vi "Process.vi"(8 "error in":errorcluster, 11 "ParseVectorFile":refnum<class "ParseVectorFile.lvclass">) -> (0 "error out":errorcluster, 3 "ParseVectorFile out":refnum<class "ParseVectorFile.lvclass">)   [LabVIEW 2019, in "ParseVectorFile.lvclass"]
doc: "---------------------------------------------------------------\nJKI State Machine Objects™\nhttp://jki.net/state-machine-objects/\nCopyright (C) 2005-2015, JKI <info@jki.net>\nALL RIGHTS RESERVED"
uses:
  ParseVectorFile.lvclass
  C:/Program Files (x86)/National Instruments/LabVIEW 2019/vi.lib/JKI/JKI SMO/SMO/SMO.lvclass
  <vilib>/JKI/JKI SMO/SMO/Typedefs/Parent Call--Enum.ctl
  Typedefs/PublicEvents--ParseVectorFile.ParsedData.ctl
  ParsePaths/Path.lvclass
  Rectangle/Rectangle.lvclass
  Image/SVGImage.lvclass
  Dot/Dot.lvclass
  <vilib>/JKI/JKI SMO/SMO/SMO.lvclass/SMO.ctl
  ParseVectorFile.lvclass/ParseVectorFile.ctl
  <vilib>/JKI/JKI SMO/SMO/Private/ReftoDVR--SMO.vi
  <vilib>/JKI/JKI SMO/SMO/SMO.lvclass
panel:
  # "For instructions on how to use the JKI State Machine Objects, examples and video tutorials, visit:\nhttp://jki.net/state-machine-objects/\n\nJKI State Machine Objects™\nhttp://jki.net/state-machine-objects/\nCopyright (C) 2005-2015, JKI <info@jki.net>\nALL RIGHTS RESERVED"
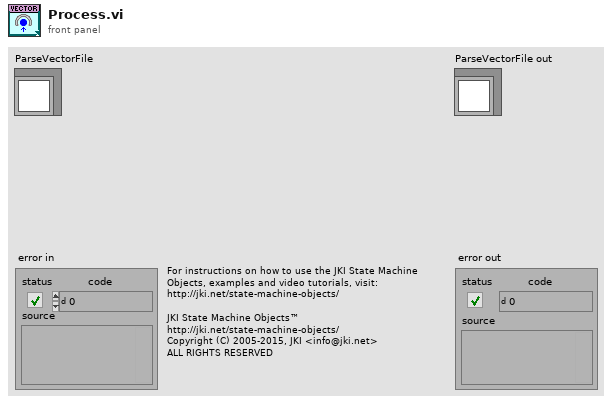
[diagram p1: front panel]
types:
  T1 = typedef "SMO.lvclass/Parent Call--Enum.ctl" = enum16{"Allows parent to run", "Does not request parent to run"}
  T2 = enum32{"invalid app kind", "Development System", "Run Time System", "Student Edition", "Embedded LabVIEW", "Evaluation", "Custom"}
  T3 = enum32{"Invalid", "Standard", "Closed", "Hidden", "Minimized", "Maximized"}
  T4 = enum32{"Bad", "Idle", "Run top level", "Running"}
  T5 = typedef "ParseVectorFile.lvclass/PublicEvents--ParseVectorFile.ParsedData.ctl" = cluster{"Paths":refnum<class "Path.lvclass">[], "Rectangles":refnum<class "Rectangle.lvclass">[], "SVGImage":refnum<class "SVGImage.lvclass">, "Dots":refnum<class "Dot.lvclass">[]}
  T6 = typedef "ParseVectorFile.lvclass/PrivateEvents--ParseVectorFile.NewFile.ctl" = path
  T7 = cluster{"Core":cluster{"Current VI Reference":refnum<vi>, "Close Panel on Exit?":bool, "error":errorcluster}, "Path":path, "Self":refnum<class "ParseVectorFile.lvclass">, "Parsed Data Return":refnum<notifier>, "Last Changed":timestamp}
  T8 = cluster{"Current VI Reference":refnum<vi>, "Close Panel on Exit?":bool, "error":errorcluster}
  T9 = typedef "SMO.lvclass/Protected Events.ctl" = cluster{"StopProcesses":refnum<user-event>, "AbortProcesses":refnum<user-event>, "Config Changed":refnum<user-event>, "Dependency":refnum<user-event>}
  T10 = typedef "ParseVectorFile.lvclass/PrivateEvents--Cluster.ctl" = cluster{"NewFile Asynchronous":refnum<user-event>, "New File Synchronous":refnum<user-event>}
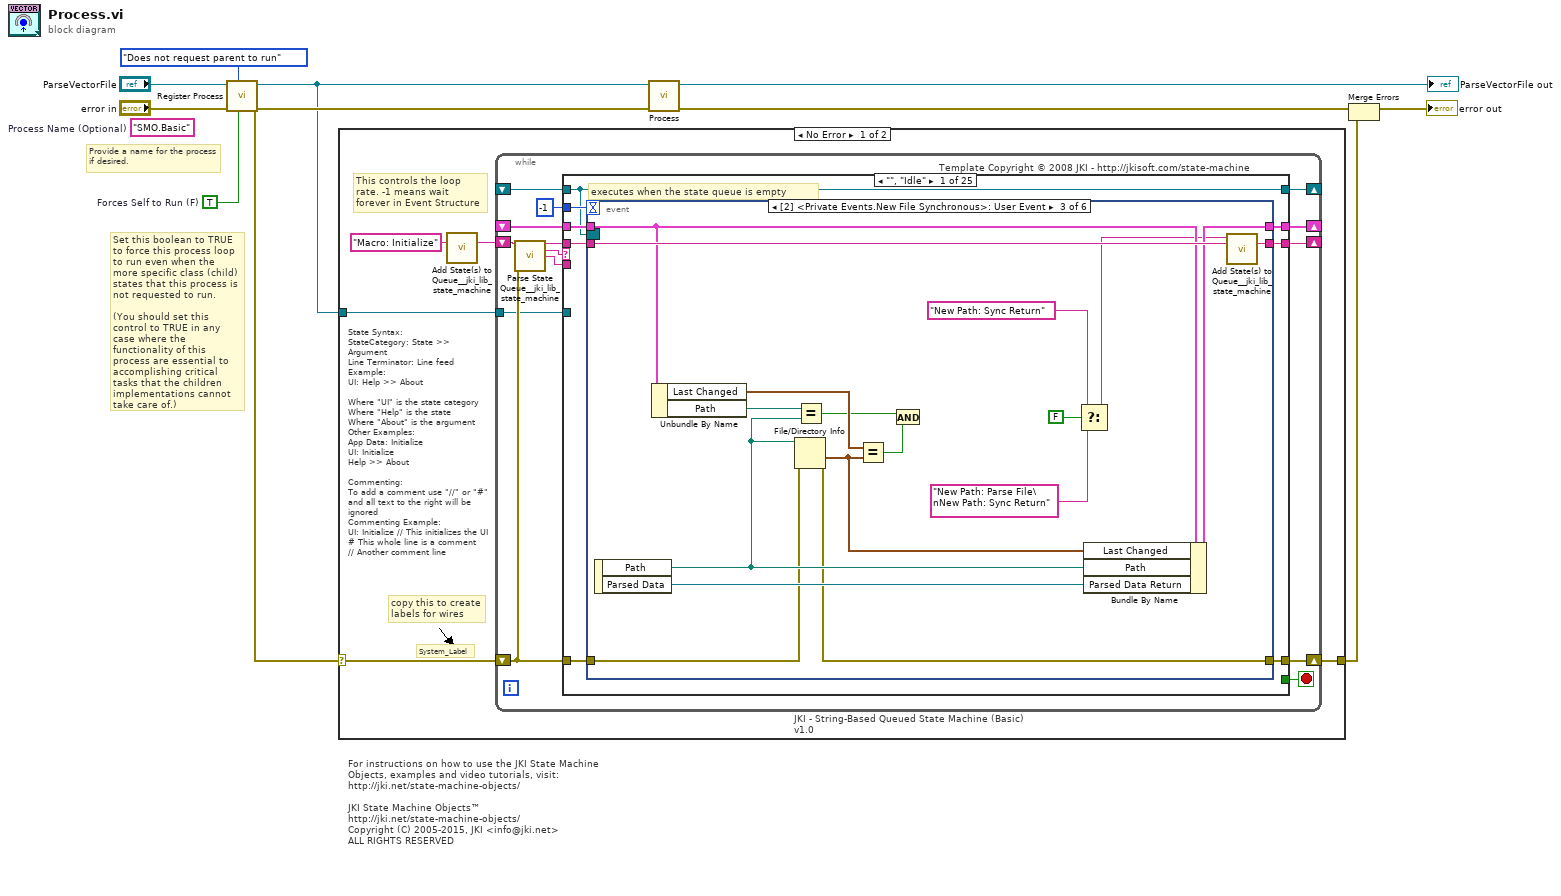
[diagram p0: block diagram]
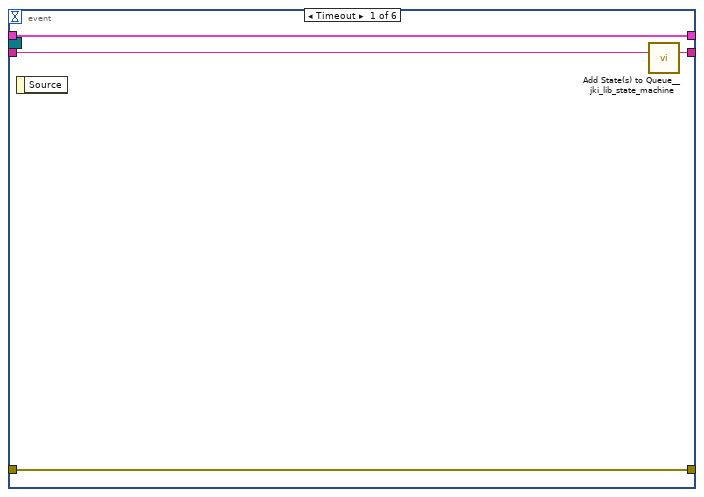
[diagram p2: hidden frame]
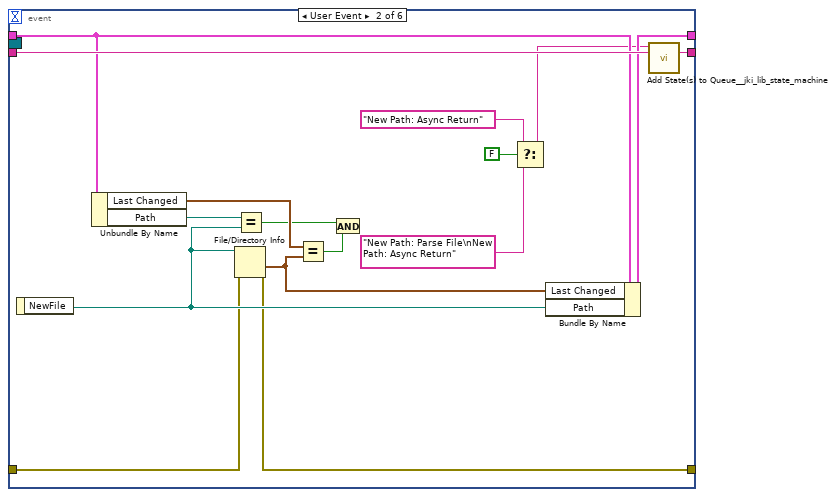
[diagram p3: hidden frame]
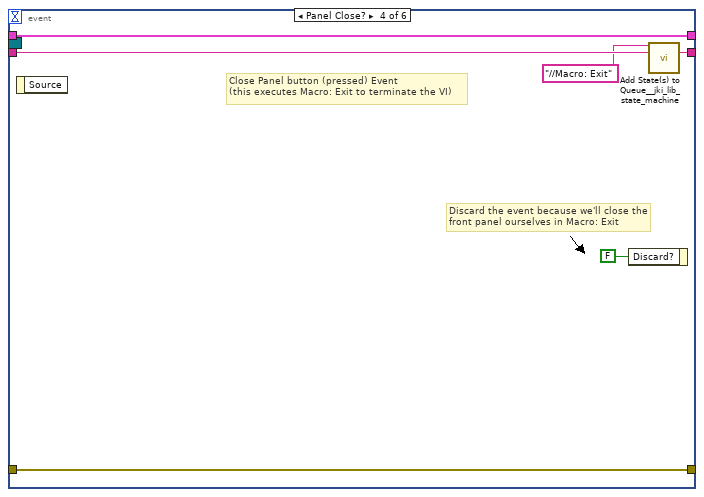
[diagram p4: hidden frame]
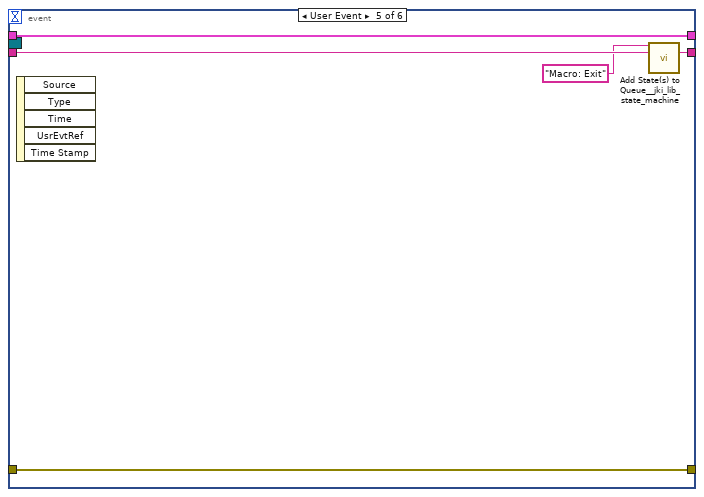
[diagram p5: hidden frame]
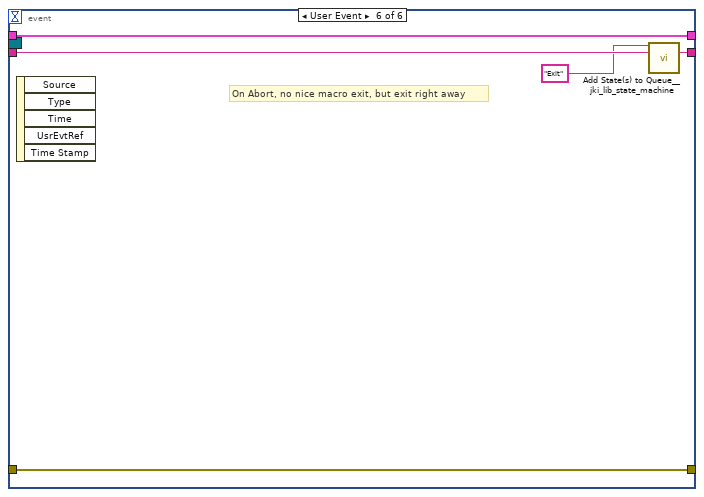
[diagram p6: hidden frame]
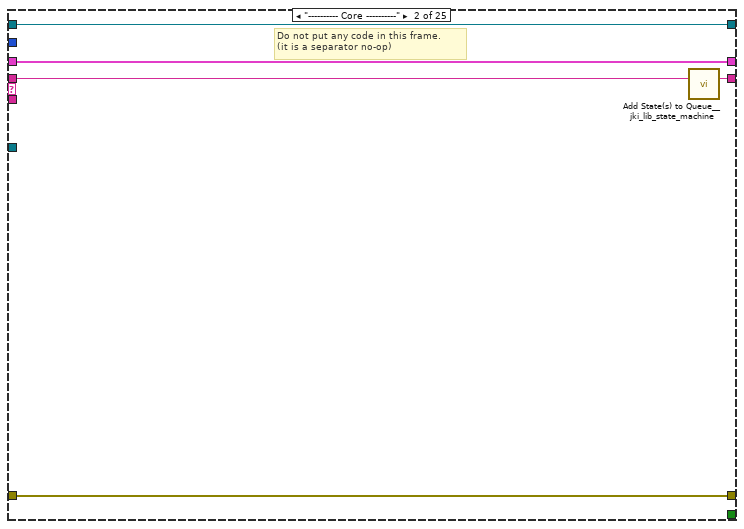
[diagram p7: hidden frame]
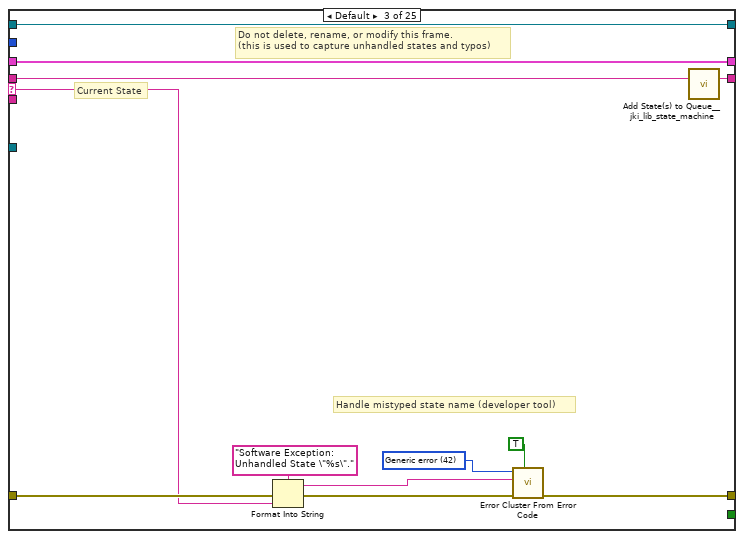
[diagram p8: hidden frame]
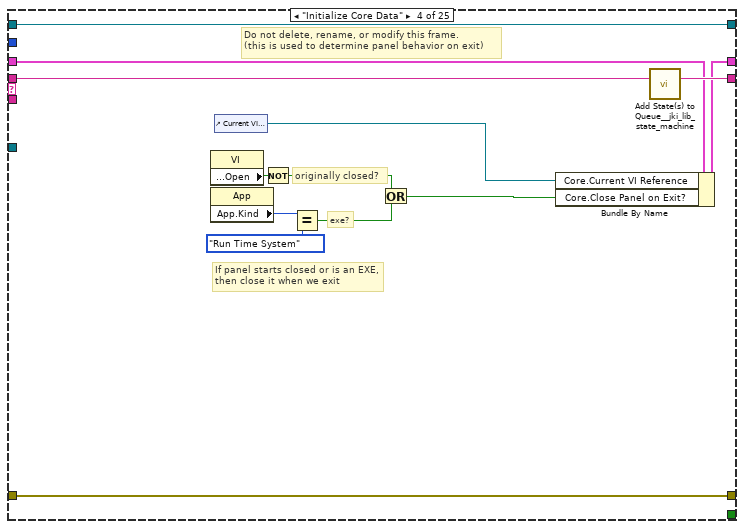
[diagram p9: hidden frame]
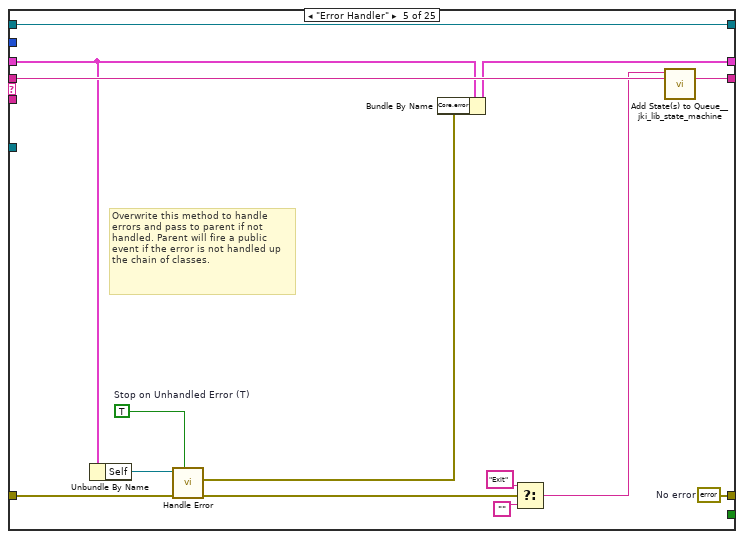
[diagram p10: hidden frame]
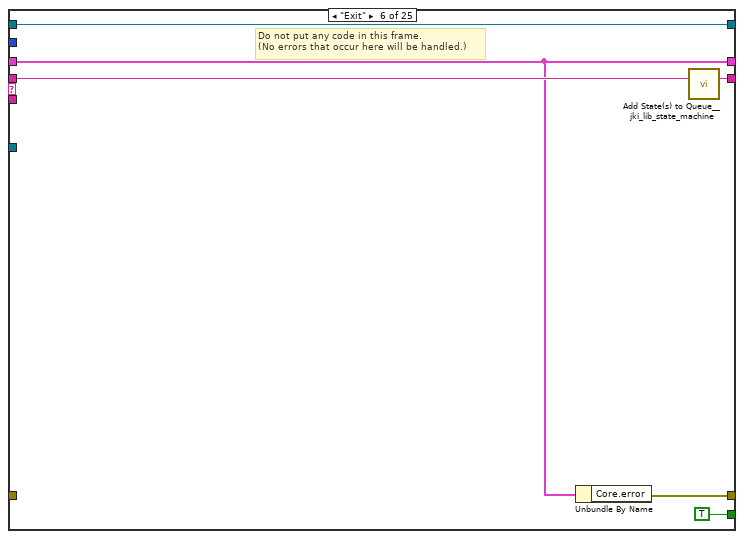
[diagram p11: hidden frame]
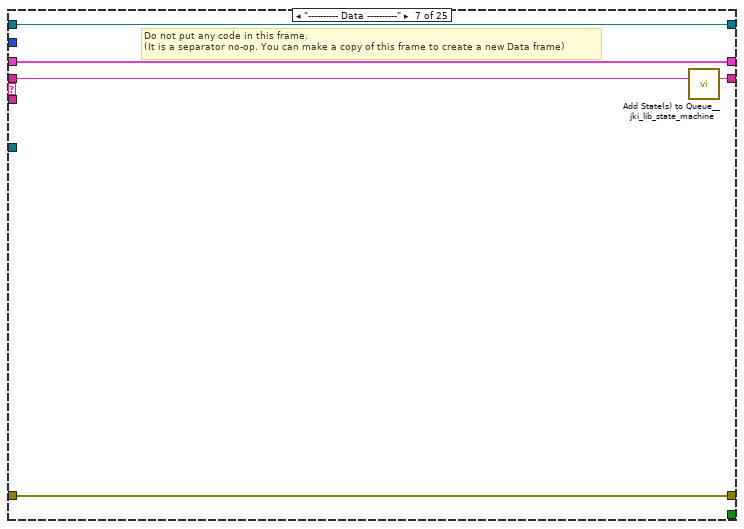
[diagram p12: hidden frame]
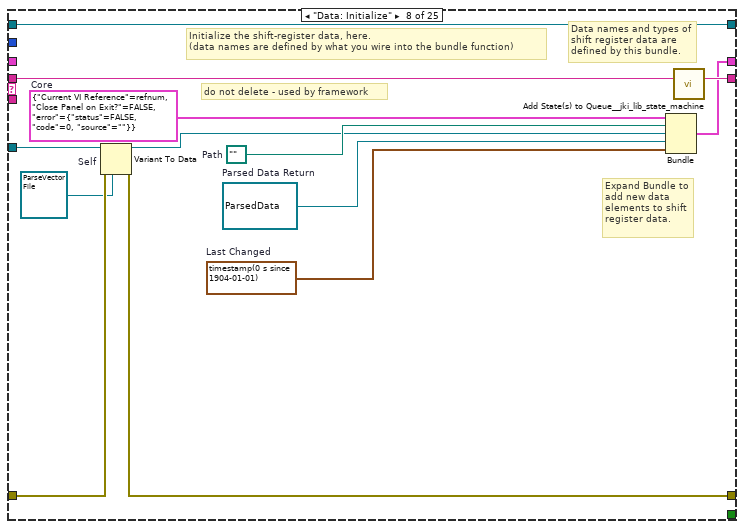
[diagram p13: hidden frame]
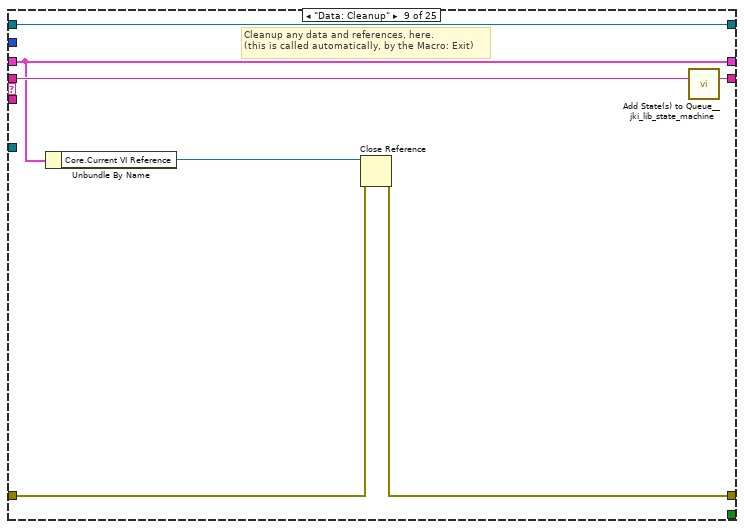
[diagram p14: hidden frame]
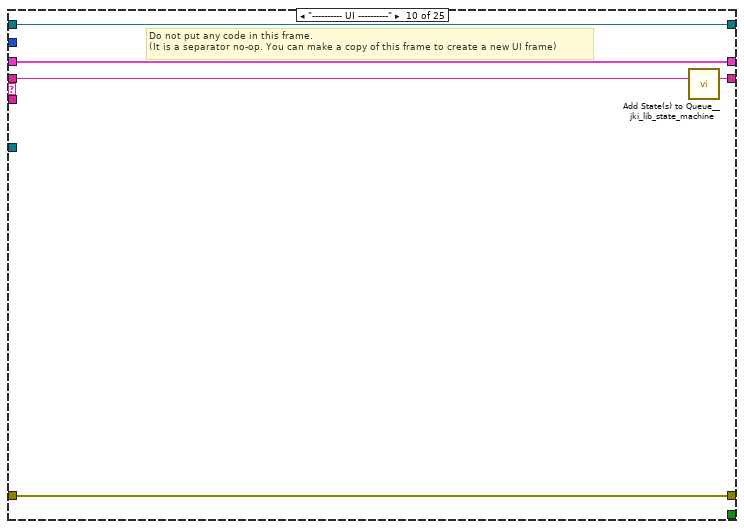
[diagram p15: hidden frame]
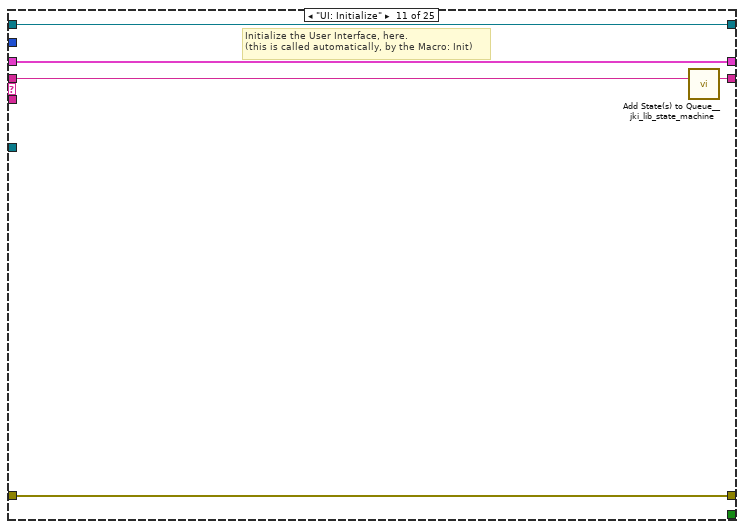
[diagram p16: hidden frame]
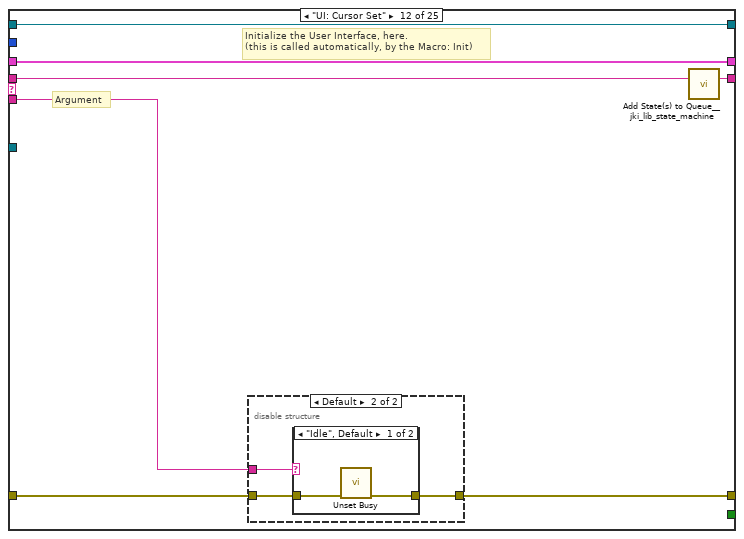
[diagram p17: hidden frame]
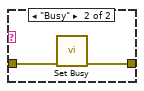
[diagram p19: hidden frame]
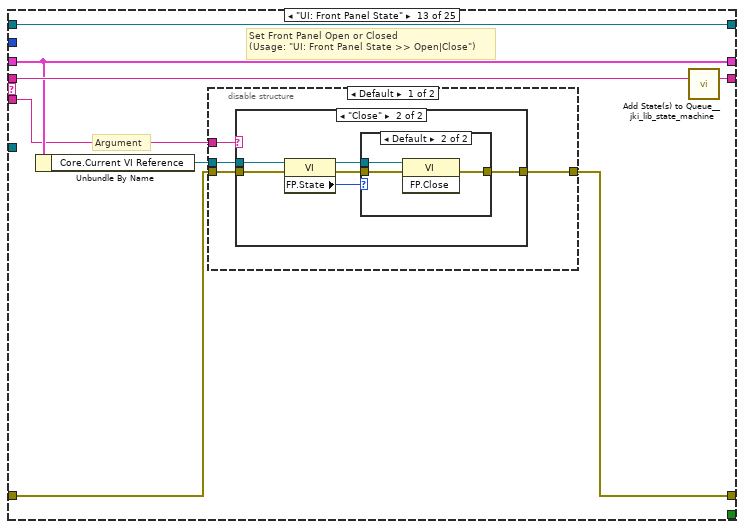
[diagram p20: hidden frame]
diagram:
  w1 = TRUE  # Forces Self to Run (F)
  (unwired) "SMO.Basic"  # Process Name (Optional)
  # "Provide a name for the process\nif desired."
  # "Set this boolean to TRUE to force this process loop to run even when the more specific class (child) states that this process is not requested to run.\n\n(You should set this control to TRUE in any case where the functionality of this process are essential to accomplishing critical tasks that the children implementations cannot take care of.)"
  # "For instructions on how to use the JKI State Machine Objects, examples and video tutorials, visit:\nhttp://jki.net/state-machine-objects/\n\nJKI State Machine Objects™\nhttp://jki.net/state-machine-objects/\nCopyright (C) 2005-2015, JKI <info@jki.net>\nALL RIGHTS RESERVED"
  n1 = call <vilib>:"Register Process.vi"("Forces Self to Run (F)"=w1, "Parent Call"=Parent_Call--Enum."Does not request parent to run", "error in (no error)"="error in", "SMO"="ParseVectorFile") -> ("error out"=w7:errorcluster, "SMO out"=w6:refnum<class "ParseVectorFile.lvclass">)  [unwired: 6 in]
  n2 = case shown="No Error" w7 {
    selector: w7 -> [w12 w345]
    tunnel: w6 -> [w13 _]
    tunnel: [w11 w345] -> w3
    frame No Error {
      # "State Syntax:\nStateCategory: State >> Argument\nLine Terminator: Line feed\nExample:\nUI: Help >> About\n\nWhere \"UI\" is the state category\nWhere \"Help\" is the state\nWhere \"About\" is the argument\nOther Examples:\nApp Data: Initialize\nUI: Initialize\nHelp >> About\n\nCommenting:\nTo add a comment use \"//\" or \"#\" and all text to the right will be ignored\nCommenting Example:\nUI: Initialize // This initializes the UI\n# This whole line is a comment\n// Another comment line"
      # "copy this to create labels for wires"
      # "This controls the loop rate. -1 means wait forever in Event Structure"
      # "System_Label"
      n3 = call <vilib>:"Add State(s) to Queue__jki_lib_state_machine.vi"("State(s) in (\"\")"="Macro: Initialize") -> ("States Out"=w15:string)  [unwired: 14 in]
      n4 = while "JKI - String-Based Queued State Machine (Basic) v1.0" {
        shift-right: [w22] -> _
        shift-left: _ -> [w21]
        shift-right: [w25] -> w11
        shift-left: w12 -> [w19]
        shift-right: [w24] -> _
        shift-left: w15 -> [w26]
        tunnel: w13 -> [w18]
        shift-right: [w17] -> _
        shift-left: _ -> [w16]
        stop <- w23 stop-if-true
        # "Template Copyright © 2008 JKI - http://jkisoft.com/state-machine"
        n5 = call <vilib>:"Parse State Queue__jki_lib_state_machine.vi"("State Queue"=w26, "Error In (no error)"=w19) -> ("Remaining States"=w28:string, "Current State"=w29:string, "Arguments"=w27:string)  [unwired: 11 in]
        n6 = case shown="\"\", \"Idle\"" w29 {
          selector: w29 -> [_ _ w97 _ _ _ _ _ _ _ _ _ _ _ _ _ _ _ _ _ _ _ _ _ _]
          tunnel: w28 -> [w37 w95 w101 w120 w134 w140 w145 w158 w165 w170 w175 w182 w198 w230 w244 w258 w263 w274 w279 w291 w297 w304 w319 w334 w344]
          tunnel: w27 -> [_ _ _ _ _ _ _ _ _ _ _ w176 w192 _ _ _ _ _ _ _ _ _ _ _ _]
          tunnel: w21 -> [w35 w92 w99 w111 w128 w136 w142 _ w160 w167 w173 w180 w194 w227 w240 w249 w260 w271 w276 w289 w295 w299 w315 w330 w341]
          tunnel: [w34 w93 w103 w117 w129 w135 w143 w154 w161 w168 w172 w177 w195 w228 w242 w256 w261 w265 w277 w285 w293 w301 w307 w322 w335] -> w25
          tunnel: w19 -> [w33 w93 w102 w117 w130 _ w143 w155 w162 w168 w172 w178 w196 w228 w242 w256 w261 w266 w277 w286 w293 w301 w307 w321 w338]
          tunnel: [w36 w94 w100 w119 w133 w139 w144 w157 w164 w169 w174 w181 w197 w229 w243 w257 w262 w273 w278 w290 w296 w303 w318 w333 w343] -> w24
          tunnel: [_ _ _ _ _ TRUE _ _ _ _ _ _ _ _ _ _ _ _ _ _ _ _ _ _ _] -> w23
          tunnel: [w32 w92 w99 w118 w127 w136 w142 w156 w160 w167 w173 w180 w194 w227 w240 w249 w260 w271 w276 w289 w295 w300 w316 w331 w340] -> w22
          tunnel: -1 ("Timeout") -> [w31 _ _ _ _ _ _ _ _ _ _ _ _ _ _ _ _ _ _ _ _ _ _ _ _]
          tunnel: w18 -> [_ _ _ _ _ _ _ w153 _ _ _ _ _ _ _ _ _ _ _ _ _ _ _ _ _]
          tunnel: [w30 w91 w96 w108 w132 w137 w141 w152 w159 w166 w171 w179 w191 w226 w241 w250 w259 w272 w275 w288 w294 w302 w317 w332 w342] -> w17
          tunnel: w16 -> [w30 w91 w96 w108 w132 w137 w141 w152 w159 w166 w171 w179 w191 w226 w241 w250 w259 w272 w275 _ w294 w302 w317 w332 w342]
          frame "", "Idle" {
            # "executes when the state queue is empty"
            n7 = event shown="[2] <Private Events.New File Synchronous>: User Event" {
              selector: w30 -> [_ _ _ _ _ _]
              dyn-events: _ -> [_ _ _ _ _ _]
              timeout: w31 -> [_ _ _ _ _ _]
              tunnel: w37 -> [w41 w57 w74 w80 w85 w90]
              tunnel: [w40 w56 w73 w79 w84 w89] -> w36
              tunnel: w35 -> [w39 w54 w65 w77 w82 w87]
              tunnel: [w38 w51 w60 w78 w83 w88] -> w34
              tunnel: w33 -> [w38 w50 w59 w78 w83 w88]
              tunnel: [w39 w55 w72 w77 w82 w87] -> w32
              event Timeout {
                n8 = event-data() -> ()  [unwired: 1 in, 1 out]
                n9 = call <vilib>:"Add State(s) to Queue__jki_lib_state_machine.vi"("State(s) in (\"\")"=w41) -> ("States Out"=w40:string)  [unwired: 14 in]
              }
              event User Event {
                n10 = event-data() -> ("NewFile"=w52:T6)  [unwired: 1 in]
                n11 = Unbundle By Name(w54) -> ("Last Changed"=w49:timestamp, "Path"=w53:path)
                n12 = File/Directory Info(path=w52, error in=w50) -> (last mod=w46:timestamp, error out=w51:errorcluster)  [unwired: 5 out]
                n13 = Equal?(x=w53, y=w52) -> (x = y?=w48:bool)
                n14 = Equal?(x=w49, y=w46) -> (x = y?=w47:bool)
                n15 = And(x=w48, y=w47) -> ()  [unwired: 1 out]
                n16 = Select(t="New Path: Async Return", s=FALSE, f="New Path: Parse File\nNew Path: Async Return") -> (s? t:f=w43:string)
                n17 = Bundle By Name(cluster=w54, "Last Changed"=w46, "Path"=w52) -> (w55:T7)
                n18 = call <vilib>:"Add State(s) to Queue__jki_lib_state_machine.vi"("State(s) in Front (\"\")"=w43, "State(s) in (\"\")"=w57) -> ("States Out"=w56:string)  [unwired: 13 in]
              }
              event User Event {
                n19 = event-data() -> ("Path"=w64:path, "Parsed Data"=w71:refnum<notifier>)  [unwired: 1 in]
                n20 = Unbundle By Name(w65) -> ("Last Changed"=w69:timestamp, "Path"=w70:path)
                n21 = File/Directory Info(path=w64, error in=w59) -> (last mod=w63:timestamp, error out=w60:errorcluster)  [unwired: 5 out]
                n22 = Equal?(x=w70, y=w64) -> (x = y?=w68:bool)
                n23 = Equal?(x=w69, y=w63) -> (x = y?=w67:bool)
                n24 = And(x=w68, y=w67) -> ()  [unwired: 1 out]
                n25 = Select(t="New Path: Sync Return", s=FALSE, f="New Path: Parse File\nNew Path: Sync Return") -> (s? t:f=w61:string)
                n26 = Bundle By Name(cluster=w65, "Last Changed"=w63, "Path"=w64, "Parsed Data Return"=w71) -> (w72:T7)
                n27 = call <vilib>:"Add State(s) to Queue__jki_lib_state_machine.vi"("State(s) in Front (\"\")"=w61, "State(s) in (\"\")"=w74) -> ("States Out"=w73:string)  [unwired: 13 in]
              }
              event Panel Close? {
                # "Discard the event because we'll close the front panel ourselves in Macro: Exit"
                # "Close Panel button (pressed) Event\n(this executes Macro: Exit to terminate the VI)"
                n28 = event-data() -> ()  [unwired: 1 in, 1 out]
                n29 = event-data("Discard?"=FALSE) -> ()  [unwired: 1 in, 1 out]
                n30 = call <vilib>:"Add State(s) to Queue__jki_lib_state_machine.vi"("State(s) in Front (\"\")"="//Macro: Exit", "State(s) in (\"\")"=w80) -> ("States Out"=w79:string)  [unwired: 13 in]
              }
              event User Event {
                n31 = event-data() -> ()  [unwired: 1 in, 5 out]
                n32 = call <vilib>:"Add State(s) to Queue__jki_lib_state_machine.vi"("State(s) in Front (\"\")"="Macro: Exit", "State(s) in (\"\")"=w85) -> ("States Out"=w84:string)  [unwired: 13 in]
              }
              event User Event {
                # "On Abort, no nice macro exit, but exit right away"
                n33 = event-data() -> ()  [unwired: 1 in, 5 out]
                n34 = call <vilib>:"Add State(s) to Queue__jki_lib_state_machine.vi"("State(s) in Front (\"\")"="Exit", "State(s) in (\"\")"=w90) -> ("States Out"=w89:string)  [unwired: 13 in]
              }
            }
          }
          frame "---------- Core ----------" {
            # "Do not put any code in this frame.\n(it is a separator no-op)"
            n35 = call <vilib>:"Add State(s) to Queue__jki_lib_state_machine.vi"("State(s) in (\"\")"=w95) -> ("States Out"=w94:string)  [unwired: 14 in]
          }
          frame Default {
            w106 = 42 items=["No error", "Argument error", "Memory is full", "Out of zone", "End of file", "File already open", "Generic file I/O error", "File not found", "File permission error", "Disk is full", "Duplicate path", "Too many files open", "System feature not enabled", "Resource file not found", "Cannot add resource", "Resource not found", "Image not found", "Image memory error", "Pen does not exist", "Config type invalid", "Config token not found", "Config parse error", "Config memory error", "Bad external code format", "Bad external code offset", "External code not present", "Null window", "Destroy window error", "Null menu", "Print aborted", "Bad print record", "Print driver error", "Windows error during printing", "Memory error during printing", "Print dialog error", "Generic print error", "Invalid device refnum", "Device not found", "Device parameter error", "Device unit error", "Cannot open device", "Device call aborted", "Generic error", "Cancelled by user", "Object ID too low", "Object ID too high", "Object not in heap", "Unknown heap", "Unknown object (invalid DefProc)", "Unknown object (DefProc not in table)", "Message out of range", "Invalid (null) method", "Unknown message", "Manager call not supported", "Bad address", "Network operation in progress", "Network operation timed out", "Connection is busy", "Network attribute not supported", "Network error", "Address in use", "System out of memory", "Connection aborted", "Connection refused", "Not connected", "Already connected", "Connection closed", "Initialization error (interapplication manager)", "Bad occurrence", "Wait on unbound occurrence handler", "Occurrence queue overflow", "Datalog type conflict", "Unused", "Unrecognized type (interapplication manager)", "Memory corrupt", "Failed to make temporary DLL", "Old CIN version", "Drag socket not found", "Failed to load drop-object", "Failed to register OLE object", "Failed to release OLE object", "Format specifier type mismatch", "Unknown format specifier", "Too few format specifiers", "Too many format specifiers", "Scan failed", "Newer CIN version", "Error converting to variant", "Runtime menu error", "Password tampered", "Variant attribute not found", "Incompatible variant data type", "Event data is not available", "Event Store is not present", "Occurrence is not found", "Event Queue is not created", "Event info is not available", "Refnum passed is NULL", "Error retrieving Class GUID", "Error retrieving CoClass GUID", "Error retrieving TypeLib GUID.", "Bad built application magic bytes.", "Specific driver is different from the specific driver associated with the Logical Name.", "There is no session opened to the class driver.", "Max Error", "MAX - Error with config objects", "MAX - Error loading configuration", "MAX - Group not supported"]
            # "Current State"
            # "Do not delete, rename, or modify this frame.\n(this is used to capture unhandled states and typos)"
            # "Handle mistyped state name (developer tool)"
            n36 = Format Into String(format string="Software Exception: Unhandled State \"%s\"." ("message"), error in=w102, w97) -> (resulting string=w105:string, error out=w104:errorcluster)  [unwired: 1 in]
            n37 = call <vilib>:"Error Cluster From Error Code.vi"("show call chain? (False)"=TRUE, "error in (no error)"=w104, "error message (\"\")"=w105, "error code (0)"=w106) -> ("error out"=w103:errorcluster)  [unwired: 5 in]
            n38 = call <vilib>:"Add State(s) to Queue__jki_lib_state_machine.vi"("State(s) in (\"\")"=w101) -> ("States Out"=w100:string)  [unwired: 14 in]
          }
          frame "Initialize Core Data" {
            # "Do not delete, rename, or modify this frame.\n(this is used to determine panel behavior on exit)"
            # "originally closed?"
            # "exe?"
            # "If panel starts closed or is an EXE, then close it when we exit"
            n39 = property class="VI"() -> ("Front Panel.Open"=w116:bool)  [unwired: 2 in, 2 out]
            n40 = property class="App"() -> ("App.Kind"=w115:T2)  [unwired: 2 in, 2 out]
            n41 = control-ref of="Current VI Reference"() -> (w109:refnum<vi>)
            n42 = Not(x=w116) -> (.not. x?=w113:bool)
            n43 = Equal?(x=w115, y=T2."Run Time System" ("Application:Kind")) -> (x = y?=w112:bool)
            n44 = Or(x=w113, y=w112) -> (x .or. y?=w110:bool)
            n45 = Bundle By Name(cluster=w111, "Core.Current VI Reference"=w109, "Core.Close Panel on Exit?"=w110) -> (w118:T7)
            n46 = call <vilib>:"Add State(s) to Queue__jki_lib_state_machine.vi"("State(s) in (\"\")"=w120) -> ("States Out"=w119:string)  [unwired: 14 in]
          }
          frame "Error Handler" {
            w121 = TRUE  # Stop on Unhandled Error (T)
            w129 = errorcluster {"status"=FALSE, "code"=0, "source"=""}  # No error
            # "Overwrite this method to handle errors and pass to parent if not handled. Parent will fire a public event if the error is not handled up the chain of classes."
            n47 = Unbundle By Name(w128) -> ("Self"=w131:refnum<class "ParseVectorFile.lvclass">)
            n48 = call-dynamic "Handle Error.vi"("Stop on Unhandled Error (T)"=w121, "error in"=w130, "SMO"=w131) -> ("handling error"=w122:errorcluster, "Unhandled error"=w125:errorcluster)  [unwired: 6 in, 1 out]
            n49 = Bundle By Name(cluster=w128, "Core.error"=w125) -> (w127:T7)
            n50 = Select(t="Exit", s=w122, f="") -> (s? t:f=w126:string)
            n51 = call <vilib>:"Add State(s) to Queue__jki_lib_state_machine.vi"("State(s) in Front (\"\")"=w126, "State(s) in (\"\")"=w134) -> ("States Out"=w133:string)  [unwired: 13 in]
          }
          frame "Exit" {
            # "Do not put any code in this frame.\n(No errors that occur here will be handled.)"
            n52 = Unbundle By Name(w136) -> ("Core.error"=w135:errorcluster)
            n53 = call <vilib>:"Add State(s) to Queue__jki_lib_state_machine.vi"("State(s) in (\"\")"=w140) -> ("States Out"=w139:string)  [unwired: 14 in]
          }
          frame "---------- Data ----------" {
            # "Do not put any code in this frame.\n(It is a separator no-op. You can make a copy of this frame to create a new Data frame)"
            n54 = call <vilib>:"Add State(s) to Queue__jki_lib_state_machine.vi"("State(s) in (\"\")"=w145) -> ("States Out"=w144:string)  [unwired: 14 in]
          }
          frame "Data: Initialize" {
            w146 = timestamp(0 s since 1904-01-01)  # Last Changed
            w149 = refnum<notifier> refnum  # Parsed Data Return
            w150 = path ""  # Path
            w151 = T8 {"Current VI Reference"=refnum, "Close Panel on Exit?"=FALSE, "error"={"status"=FALSE, "code"=0, "source"=""}}  # Core
            w148 = refnum<class "ParseVectorFile.lvclass"> refnum  # Self
            # "do not delete - used by framework"
            # "Expand Bundle to add new data elements to shift register data."
            # "Data names and types of shift register data are defined by this bundle."
            # "Initialize the shift-register data, here.\n(data names are defined by what you wire into the bundle function)"
            n55 = Variant To Data(error in=w155, type=w148, Variant=w153) -> (data=w147:refnum<class "ParseVectorFile.lvclass">, error out=w154:errorcluster)
            n56 = Bundle("Core"=w151, "Path"=w150, "Self"=w147, "Parsed Data Return"=w149, "Last Changed"=w146) -> (w156:T7)  [unwired: 1 in]
            n57 = call <vilib>:"Add State(s) to Queue__jki_lib_state_machine.vi"("State(s) in (\"\")"=w158) -> ("States Out"=w157:string)  [unwired: 14 in]
          }
          frame "Data: Cleanup" {
            # "Cleanup any data and references, here.\n(this is called automatically, by the Macro: Exit)"
            n58 = Unbundle By Name(w160) -> ("Core.Current VI Reference"=w163:refnum<vi>)
            n59 = Close Reference(reference=w163, error in (no error)=w162) -> (error out=w161:errorcluster)
            n60 = call <vilib>:"Add State(s) to Queue__jki_lib_state_machine.vi"("State(s) in (\"\")"=w165) -> ("States Out"=w164:string)  [unwired: 14 in]
          }
          frame "---------- UI ----------" {
            # "Do not put any code in this frame.\n(It is a separator no-op. You can make a copy of this frame to create a new UI frame)"
            n61 = call <vilib>:"Add State(s) to Queue__jki_lib_state_machine.vi"("State(s) in (\"\")"=w170) -> ("States Out"=w169:string)  [unwired: 14 in]
          }
          frame "UI: Initialize" {
            # "Initialize the User Interface, here.\n(this is called automatically, by the Macro: Init)"
            n62 = call <vilib>:"Add State(s) to Queue__jki_lib_state_machine.vi"("State(s) in (\"\")"=w175) -> ("States Out"=w174:string)  [unwired: 14 in]
          }
          frame "UI: Cursor Set" {
            # "Argument"
            # "Initialize the User Interface, here.\n(this is called automatically, by the Macro: Init)"
            n63 = disable-structure shown="Default" {
              disable-tunnel: w178 -> [w183 w186]
              disable-tunnel: [w183 w185] -> w177
              disable-tunnel: w176 -> [_ w184]
              frame condition #0 {
              }
              frame condition #1 (active) {
                n64 = case shown="\"Idle\", Default" w184 {
                  tunnel: w186 -> [w188 w190]
                  tunnel: [w187 w189] -> w185
                  frame "Idle", Default {
                    n65 = call <vilib>:"Unset Busy.vi"("error in (no error)"=w188) -> ("error out"=w187:errorcluster)  [unwired: 10 in]
                  }
                  frame "Busy" {
                    n66 = call <vilib>:"Set Busy.vi"("error in (no error)"=w190) -> ("error out"=w189:errorcluster)  [unwired: 9 in, 1 out]
                  }
                }
              }
            }
            n67 = call <vilib>:"Add State(s) to Queue__jki_lib_state_machine.vi"("State(s) in (\"\")"=w182) -> ("States Out"=w181:string)  [unwired: 14 in]
          }
          frame "UI: Front Panel State" {
            # "Argument"
            # "Set Front Panel Open or Closed\n(Usage: \"UI: Front Panel State >> Open|Close\")"
            n68 = Unbundle By Name(w194) -> ("Core.Current VI Reference"=w193:refnum<vi>)
            n69 = disable-structure shown="Default" {
              disable-tunnel: w196 -> [w202 w225]
              disable-tunnel: [w201 w225] -> w195
              disable-tunnel: w193 -> [w200 _]
              disable-tunnel: w192 -> [w199 _]
              frame condition #0 (active) {
                n70 = case shown="\"Close\"" w199 {
                  tunnel: w202 -> [w206 w219]
                  tunnel: [w208 w220] -> w201
                  tunnel: w200 -> [w207 w217]
                  frame "Open", Default {
                    n71 = property class="VI"(reference=w207, error in=w206) -> (reference out=w204:refnum<vi>, error out=w205:errorcluster, "FP.State"=w203:T3)
                    n72 = case shown="\"Closed\"" w203 {
                      tunnel: [w211 w214] -> w208
                      tunnel: w205 -> [w210 w214]
                      tunnel: w204 -> [w209 _]
                      frame "Closed" {
                        n73 = invoke class="VI" method="FP.Open"(reference=w209, error in=w210, "Activate"=TRUE, "State"=T3."Standard") -> (error out=w211:errorcluster)  [unwired: 1 in, 4 out]
                      }
                      frame Default {
                      }
                    }
                  }
                  frame "Close" {
                    n74 = property class="VI"(reference=w217, error in=w219) -> (reference out=w216:refnum<vi>, error out=w218:errorcluster, "FP.State"=w215:T3)
                    n75 = case shown="Default" w215 {
                      tunnel: [w221 w224] -> w220
                      tunnel: w218 -> [w221 w223]
                      tunnel: w216 -> [_ w222]
                      frame "Invalid", "Closed" {
                      }
                      frame Default {
                        n76 = invoke class="VI" method="FP.Close"(reference=w222, error in=w223) -> (error out=w224:errorcluster)  [unwired: 1 in, 2 out]
                      }
                    }
                  }
                }
              }
              frame condition #1 {
              }
            }
            n77 = call <vilib>:"Add State(s) to Queue__jki_lib_state_machine.vi"("State(s) in (\"\")"=w198) -> ("States Out"=w197:string)  [unwired: 14 in]
          }
          frame "---------- Macro ----------" {
            # "Do not put any code in this frame.\n(It is a separator no-op. You can make a copy of this frame to create a new Macro frame)"
            n78 = call <vilib>:"Add State(s) to Queue__jki_lib_state_machine.vi"("State(s) in (\"\")"=w230) -> ("States Out"=w229:string)  [unwired: 14 in]
          }
          frame "Macro: Initialize" {
            w235 = "//UI: Initialize\n//UI: Front Panel State >> Open"  # //UI: Initialize //UI: Front Panel State >> Open
            w231 = "Process: Sync"
            # "Initialization Macro\n(This is called once, when the VI starts)"
            n79 = control-ref of="This VI"() -> (w233:refnum<vi>)
            n80 = property class="VI"(reference=w233) -> ("Exec.State"=w232:T4)  [unwired: 1 in, 2 out]
            n81 = Equal?(x=w232, y=T4."Run top level") -> (x = y?=w238:bool)
            n82 = Select(t=w231, s=w238, f="") -> ()  [unwired: 1 out]
            n83 = call <vilib>:"Add State(s) to Queue__jki_lib_state_machine.vi"("State(s) in Front (\"\")"="Data: Initialize\nInitialize Core Data\nEvents: Register", "State(s) in (\"\")"=w231, "State(s) at Back (\"\")"=w235) -> ("States Out"=w234:string)  [unwired: 12 in]
            n84 = call <vilib>:"Add State(s) to Queue__jki_lib_state_machine.vi"("State(s) in Front (\"\")"=w234, "State(s) in (\"\")"=w244) -> ("States Out"=w243:string)  [unwired: 13 in]
          }
          frame "Macro: Exit" {
            # "Exit Macro\n(This is called once, when the VI exits)"
            n85 = Unbundle By Name(w249) -> ("Core.Close Panel on Exit?"=w255:bool)
            n86 = Select(t="UI: Front Panel State >> Close", s=w255, f="") -> (s? t:f=w252:string)
            n87 = call <vilib>:"Add State(s) to Queue__jki_lib_state_machine.vi"("State(s) in Front (\"\")"="Data: Cleanup\nEvents: Unregister", "State(s) in (\"\")"="Process: Sync", "State(s) at Back (\"\")"="Exit") -> ("States Out"=w246:string)  [unwired: 12 in]
            n88 = call <vilib>:"Add State(s) to Queue__jki_lib_state_machine.vi"("State(s) in (\"\")"=w252, "State(s) at Back (\"\")"=w246) -> ("States Out"=w251:string)  [unwired: 13 in]
            n89 = call <vilib>:"Add State(s) to Queue__jki_lib_state_machine.vi"("State(s) in Front (\"\")"=w251, "State(s) in (\"\")"=w258) -> ("States Out"=w257:string)  [unwired: 13 in]
          }
          frame "---------- Process ----------" {
            # "Template Separator\n(You can make a copy of, or modify, this frame)"
            n90 = call <vilib>:"Add State(s) to Queue__jki_lib_state_machine.vi"("State(s) in (\"\")"=w263) -> ("States Out"=w262:string)  [unwired: 14 in]
          }
          frame "Process: Sync" {
            n91 = Unbundle By Name(w271) -> ("Self"=w267:refnum<class "ParseVectorFile.lvclass">)
            n92 = call <vilib>:"WaitOnProcessSync.vi"("error in (no error)"=w266, "SMO"=w267) -> ("error out"=w265:errorcluster, "Don't run?"=w270:bool)  [unwired: 7 in, 1 out]
            n93 = Select(t="Data: Cleanup\nEvents: Unregister\nExit", s=w270, f="") -> (s? t:f=w264:string)
            n94 = call <vilib>:"Add State(s) to Queue__jki_lib_state_machine.vi"("State(s) in Front (\"\")"=w264, "State(s) in (\"\")"=w274) -> ("States Out"=w273:string)  [unwired: 13 in]
          }
          frame "---------- Events ----------" {
            # "Template Separator\n(You can make a copy of, or modify, this frame)"
            n95 = call <vilib>:"Add State(s) to Queue__jki_lib_state_machine.vi"("State(s) in (\"\")"=w279) -> ("States Out"=w278:string)  [unwired: 14 in]
          }
          frame "Events: Register" {
            # "Expand to add\nmore events"
            n96 = Unbundle By Name(w289) -> ("Self"=w282:refnum<class "ParseVectorFile.lvclass">)
            n97 = call <vilib>:"GetProtectedEvents.vi"("SMO"=w282) -> ("error out"=w283:errorcluster, "SMO Protected Events"=w287:T9)  [unwired: 8 in, 1 out]
            n98 = call "ParseVectorFile.GetPrivateEvents.vi"("ParseVectorFile"=w282) -> ("error out"=w281:errorcluster, "Private Events"=w280:T10)  [unwired: 8 in, 1 out]
            n99 = register-events(w287, w280) -> (reference out=w288:refnum<event-registration>, error out=w284:errorcluster)  [unwired: 2 in]
            n100 = Merge Errors(w286, w284, w283, w281) -> (w285:errorcluster)
            n101 = call <vilib>:"Add State(s) to Queue__jki_lib_state_machine.vi"("State(s) in (\"\")"=w291) -> ("States Out"=w290:string)  [unwired: 14 in]
          }
          frame "Events: Unregister" {
            n102 = Unregister For Events(event registration refnum=w294, error in=w293) -> (error out=w292:errorcluster)
            n103 = call <vilib>:"Clear Errors.vi"("error in (no error)"=w292) -> ()  [unwired: 5 in, 2 out]
            n104 = call <vilib>:"Add State(s) to Queue__jki_lib_state_machine.vi"("State(s) in (\"\")"=w297) -> ("States Out"=w296:string)  [unwired: 14 in]
          }
          frame "---------- New Path ----------" {
            n105 = Unbundle By Name(w299) -> ("Path"=w298:path)
            n106 = Bundle By Name(cluster=w299, "Path"=w298) -> (w300:T7)
            n107 = call <vilib>:"Add State(s) to Queue__jki_lib_state_machine.vi"("State(s) in (\"\")"=w304) -> ("States Out"=w303:string)  [unwired: 14 in]
          }
          frame "New Path: Sync Return" {
            n108 = Unbundle By Name(w315) -> ("Parsed Data Return"=w309:refnum<notifier>, "Self"=w306:refnum<class "ParseVectorFile.lvclass">)
            n109 = Unbundle By Name(w306) -> ("Paths"=w313:refnum<class "Path.lvclass">[], "Rectangles"=w312:refnum<class "Rectangle.lvclass">[], "SVGImage"=w311:refnum<class "SVGImage.lvclass">, "Dots"=w305:refnum<class "Dot.lvclass">[])
            n110 = Bundle By Name(cluster=T5 {"Paths"=[], "Rectangles"=[], "SVGImage"=refnum, "Dots"=[]} ("ParsedData"), "Paths"=w313, "Rectangles"=w312, "SVGImage"=w311, "Dots"=w305) -> (w310:T5)
            n111 = Send Notification(notification=w310, notifier=w309) -> (error out=w308:errorcluster)  [unwired: 1 in, 1 out]
            n112 = call <vilib>:"Clear Errors.vi"("error in (no error)"=w308) -> ()  [unwired: 5 in, 2 out]
            n113 = Bundle By Name(cluster=w315, "Self"=w306) -> (w316:T7)
            n114 = call <vilib>:"Add State(s) to Queue__jki_lib_state_machine.vi"("State(s) in (\"\")"=w319) -> ("States Out"=w318:string)  [unwired: 14 in]
          }
          frame "New Path: Async Return" {
            n115 = Unbundle By Name(w330) -> ("Self"=w324:refnum<class "ParseVectorFile.lvclass">)
            n116 = Unbundle By Name(w324) -> ("Paths"=w327:refnum<class "Path.lvclass">[], "Rectangles"=w326:refnum<class "Rectangle.lvclass">[], "SVGImage"=w325:refnum<class "SVGImage.lvclass">, "Dots"=w320:refnum<class "Dot.lvclass">[])
            n117 = Bundle By Name(cluster=T5 {"Paths"=[], "Rectangles"=[], "SVGImage"=refnum, "Dots"=[]} ("ParsedData"), "Paths"=w327, "Rectangles"=w326, "SVGImage"=w325, "Dots"=w320) -> (w323:T5)
            n118 = call "ParseVectorFile.ParsedData.vi"("error in (no error)"=w321, "ParsedData"=w323, "ParseVectorFile"=w324) -> ("error out"=w322:errorcluster, "ParseVectorFile out"=w329:refnum<class "ParseVectorFile.lvclass">)  [unwired: 7 in]
            n119 = Bundle By Name(cluster=w330, "Self"=w329) -> (w331:T7)
            n120 = call <vilib>:"Add State(s) to Queue__jki_lib_state_machine.vi"("State(s) in (\"\")"=w334) -> ("States Out"=w333:string)  [unwired: 14 in]
          }
          frame "New Path: Parse File" {
            n121 = Unbundle By Name(w341) -> ("Self"=w339:refnum<class "ParseVectorFile.lvclass">, "Path"=w337:path)
            n122 = call "ParseVectorFile.ParseSVG.vi"("error in (no error)"=w338, "Path"=w337, "ParseVectorFile in"=w339) -> ("error out"=w335:errorcluster, "ParseVectorFile out"=w336:refnum<class "ParseVectorFile.lvclass">)  [unwired: 7 in]
            n123 = Bundle By Name(cluster=w341, "Self"=w336) -> (w340:T7)
            n124 = call <vilib>:"Add State(s) to Queue__jki_lib_state_machine.vi"("State(s) in (\"\")"=w344) -> ("States Out"=w343:string)  [unwired: 14 in]
          }
        }
      }
    }
    frame Error {
    }
  }
  n125 = call-parent "Process.vi"("error in"=w7, "SMO"=w6) -> ("error out"=w4:errorcluster, "SMO out"=→"ParseVectorFile out":refnum<class "ParseVectorFile.lvclass">)  [unwired: 8 in]
  n126 = Merge Errors(w4, w3) -> (→"error out":errorcluster)
